vi "plot_stressXstrain.vi"(8 "error in":errorcluster, 11 "FGV_data":T1) -> (0 "error out":errorcluster, 3 "FGV_data_out":T1)   [LabVIEW 2016]
uses:
  MainFGV/FGV_data.ctl
  TypeDefs/specimen_data.ctl
  TypeDefs/specimen_info.ctl
  <vilib>/Analysis/1siggen.llb/Ramp Pattern by Samples.vi
  <vilib>/Analysis/baseanly.llb/Mean (DBL).vi
  <vilib>/Analysis/NI_AALBase.lvlib
  <vilib>/gmath/NI_Gmath.lvlib
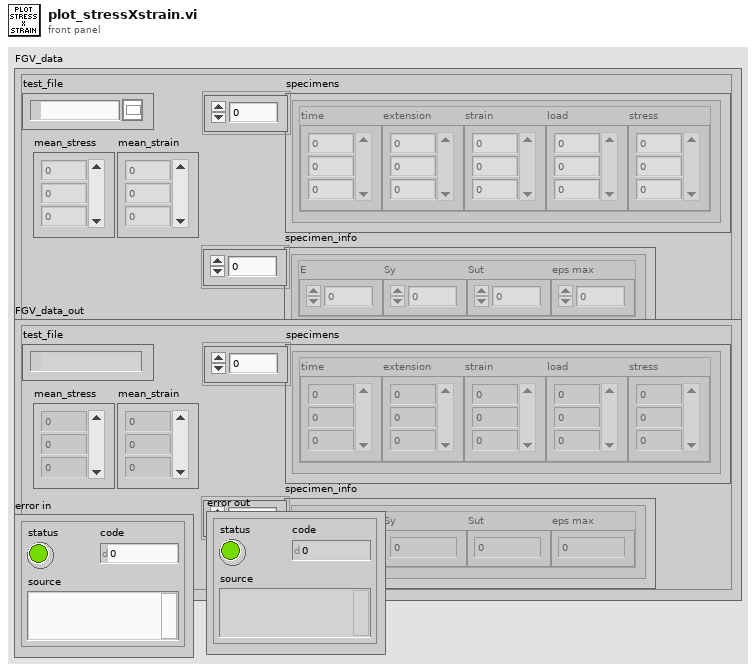
[diagram p1: front panel]
types:
  T1 = typedef "FGV_data.ctl" = cluster{"test_file":path, "specimens":T2[], "mean_strain":dbl[], "mean_stress":dbl[], "specimen_info":T3[]}
  T2 = typedef "specimen_data.ctl" = cluster{"time":dbl[], "extension":dbl[], "strain":dbl[], "load":dbl[], "stress":dbl[]}
  T3 = typedef "specimen_info.ctl" = cluster{"E":dbl, "Sy":dbl, "Sut":dbl, "eps max":dbl}
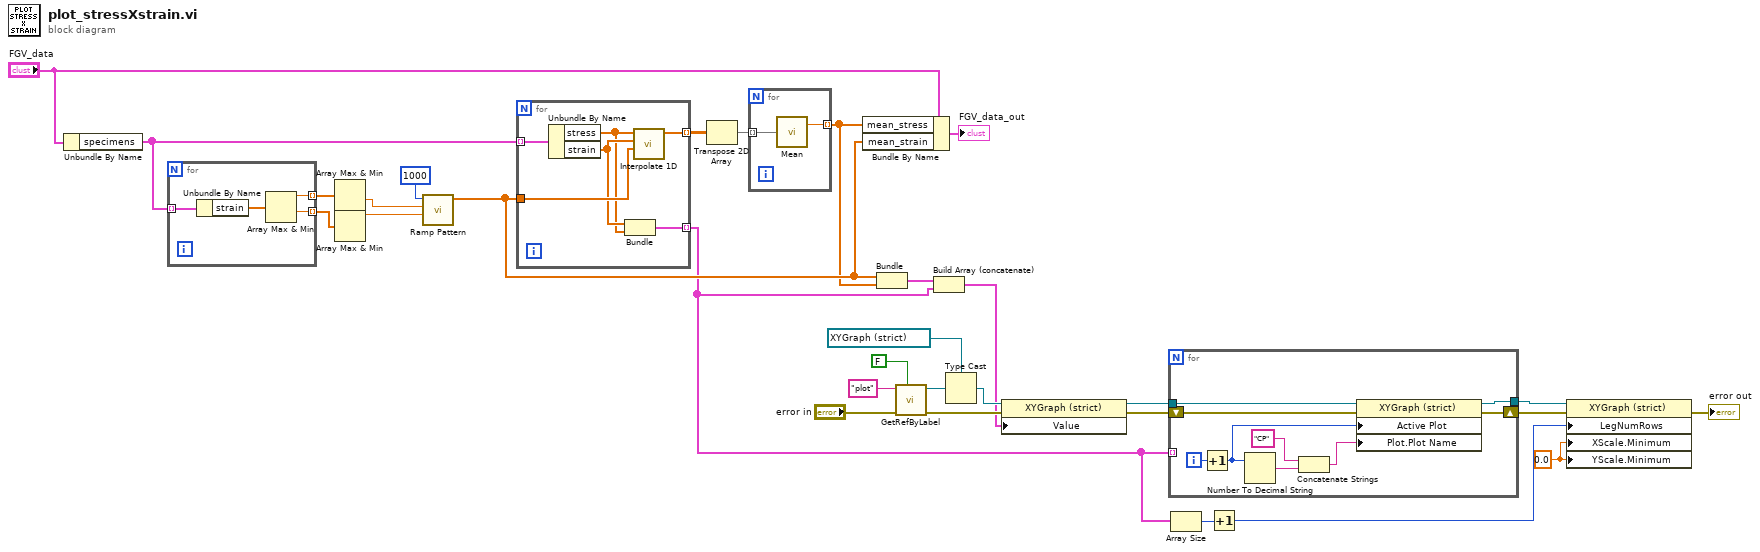
[diagram p0: block diagram]
diagram:
  w1 = 0.0 ("Y Scale.Range:Minimum")
  n1 = Unbundle By Name("FGV_data") -> ("specimens"=w25:T2[])
  n2 = for {
    tunnel: w25 -> [w34] mode=indexing
    tunnel: [w32] -> w30 mode=indexing
    tunnel: [w31] -> w29 mode=indexing
    n3 = Unbundle By Name(w34) -> ("strain"=w33:dbl[])
    n4 = Array Max & Min(array=w33) -> (max value=w32:dbl, min value=w31:dbl)  [unwired: 2 out]
  }
  n5 = Array Max & Min(array=w30) -> (min value=w27:dbl)  [unwired: 3 out]
  n6 = Array Max & Min(array=w29) -> (max value=w28:dbl)  [unwired: 3 out]
  n7 = call-poly <vilib>:"Ramp Pattern.vi"("start"=w28, "end"=w27, "samples"=1000) -> ("Ramp Pattern"=w19:dbl[])  [unwired: 7 in, 1 out]
  n8 = for {
    tunnel: w25 -> [w40] mode=indexing
    tunnel: w19 -> [w39]
    tunnel: [w38] -> w24 mode=indexing
    tunnel: [w35] -> w5 mode=indexing
    n9 = Unbundle By Name(w40) -> ("stress"=w36:dbl[], "strain"=w37:dbl[])
    n10 = Bundle("strain"=w37, "stress"=w36) -> (w35:cluster{"strain":dbl[], "stress":dbl[]})  [unwired: 1 in]
    n11 = call <vilib>:"Interpolate 1D.vi"("xi"=w39, "X"=w37, "Y"=w36) -> ("yi"=w38:dbl[])  [unwired: 6 in, 2 out]
  }
  n12 = Transpose 2D Array(2D array=w24) -> (transposed array=w23:dbl[][])
  n13 = for {
    tunnel: w23 -> [w42] mode=indexing
    tunnel: [w41] -> w18 mode=indexing
    n14 = call-poly <vilib>:"Mean.vi"("X"=w42) -> ("mean"=w41:dbl)  [unwired: 1 out]
  }
  n15 = Bundle By Name(cluster="FGV_data", "mean_stress"=w18, "mean_strain"=w19) -> (→"FGV_data_out":T1)
  n16 = Bundle("Ramp Pattern"=w19, w18) -> (w17:cluster{"Ramp Pattern":dbl[], dbl[]})  [unwired: 1 in]
  n17 = call "GetRefByLabel.vi"("InsideTab"=FALSE, "error in"="error in", "Label"="plot") -> ("error out"=w11:errorcluster, "Ctl Refnum"=w16:refnum<vi>)  [unwired: 6 in, 1 out]
  n18 = Build Array (concatenate)(w17, w5) -> (w10:cluster{"strain":dbl[], "stress":dbl[]}[])
  n19 = Type Cast(type=refnum<vi> refnum ("plot"), x=w16) -> (*(type *) &x=w12:refnum<vi>)
  n20 = property class="XYGraph (strict)"(reference=w12, error in=w11, "Value"=w10) -> (reference out=w8:refnum<vi>, error out=w9:errorcluster)
  n21 = for {
    shift-right: [w45] -> w7
    shift-left: w9 -> [w50]
    tunnel: w8 -> [w51]
    tunnel: w5 -> [_] mode=indexing
    tunnel: [w44] -> w6
    i -> [w49]
    n22 = Increment(x=w49) -> (x+1=w43:i32)
    n23 = Number To Decimal String(number=w43) -> (decimal integer string=w48:string)  [unwired: 1 in]
    n24 = Concatenate Strings("CP" ("string"), w48) -> (w46:string)
    n25 = property class="XYGraph (strict)"(reference=w51, error in=w50, "Active Plot"=w43, "Plot.Plot Name"=w46) -> (reference out=w44:refnum<vi>, error out=w45:errorcluster)
  }
  n26 = Array Size(array=w5) -> (size(s)=w4:i32)
  n27 = Increment(x=w4) -> (x+1=w2:i32)
  n28 = property class="XYGraph (strict)"(reference=w6, error in=w7, "LegNumRows"=w2, "XScale.Minimum"=w1, "YScale.Minimum"=w1) -> (error out=→"error out":errorcluster)  [unwired: 1 out]
